vi "GetAffineTransform.vi"(8 "error in":errorcluster, 10 "Dst":T1[](array[typedef]), 11 "Src":T1[](array[typedef])) -> (0 "error out":errorcluster, 3 "Result":dbl[][](array[numeric]))   [LabVIEW 2020, in "OpenLvVision_OpenCv.lvlib"]
doc: "Calculates an affine transform from three pairs of the corresponding points."
uses:
  TypeDef/Point/2D_PointSGL.ctl
  OpenLvVision_OpenCv.lvlib
  Dlls/OlvOpenCvWrapper.dll
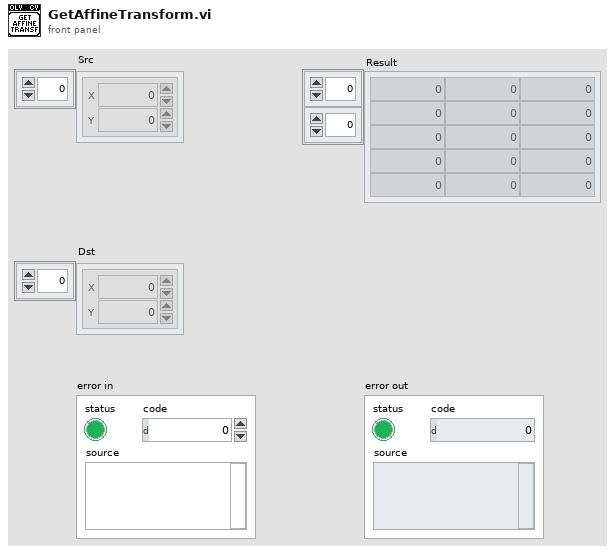
[diagram p1: front panel]
types:
  T1 = typedef "OpenLvVision_OpenCv.lvlib/2D_PointSGL.ctl" = cluster{"X":sgl, "Y":sgl}
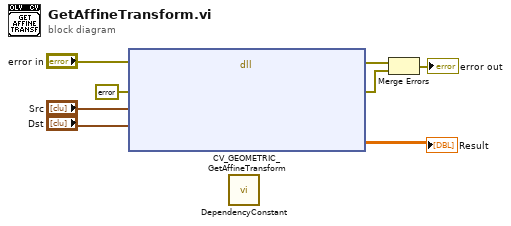
[diagram p0: block diagram]
diagram:
  n1 = dll-call lib="C:/Users/lukas/Downloads/OpenLvVision_OpenCv/SourceCode/LabView/OpenLvVision_OpenCv/Dlls/OlvOpenCvWrapper.dll" fn="CV_GEOMETRIC_GetAffineTransform"(error in="error in", "Error"=errorcluster {"status"=FALSE, "code"=0, "source"=""}, "src"="Src", "dst"="Dst") -> (error out=w6:errorcluster, "Error"=w7:errorcluster, "result"=→"Result":dbl[][])  [unwired: 6 in, 1 out]
  n2 = call "DependencyConstant.vi"() -> ()  [unwired: 12 in]
  n3 = Merge Errors(w6, w7) -> (→"error out":errorcluster)
